vi "SwerveJoystickLogic.vi"(8 "Gyro":dbl, 9 "Ackerman":bool, 10 "Joystick Axes":dbl[](array[numeric])) -> (2 "Speeds":dbl[](array[numeric]), 3 "Angles":dbl[](array[numeric]))   [LabVIEW 2018]
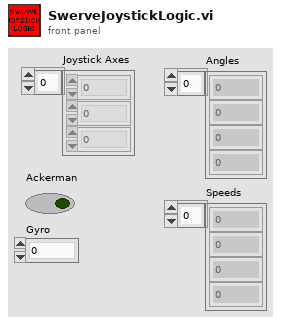
[diagram p1: front panel]
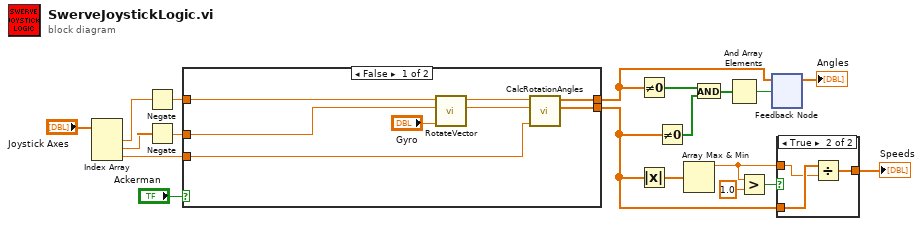
[diagram p0: block diagram]
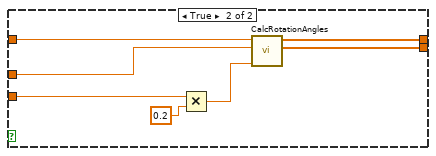
[diagram p3: hidden frame]
diagram:
  n1 = Index Array(array="Joystick Axes") -> (element #1=w6:dbl, element #2=w4:dbl, element #3=w3:dbl)  [unwired: 3 in]
  n2 = Negate(x=w6) -> (-x=w7:dbl)
  n3 = Negate(x=w4) -> (-x=w5:dbl)
  n4 = case shown="False" "Ackerman" {
    tunnel: [w27 w31] -> w14
    tunnel: w7 -> [w25 w34]
    tunnel: w5 -> [w24 w33]
    tunnel: w3 -> [w21 w29]
    tunnel: [w26 w32] -> w10
    frame False {
      n5 = call "RotateVector.vi"("Angle"="Gyro", "Y"=w24, "X"=w25) -> ("Y'"=w22:dbl, "X'"=w23:dbl)  [unwired: 6 in]
      n6 = call "CalcRotationAngles.vi"("ZAxis"=w21, "YAxis"=w22, "XAxis"=w23) -> ("Speeds"=w27:dbl[], "Angles"=w26:dbl[])  [unwired: 7 in]
    }
    frame True {
      n7 = Multiply(x=w29, y=0.2 ("x")) -> (x*y=w30:dbl)
      n8 = call "CalcRotationAngles.vi"("ZAxis"=w30, "YAxis"=w33, "XAxis"=w34) -> ("Speeds"=w31:dbl[], "Angles"=w32:dbl[])  [unwired: 7 in]
    }
  }
  n9 = Not Equal To 0?(x=w10) -> (x != 0?=w12:bool[])
  n10 = Absolute Value(x=w14) -> (abs(x)=w16:dbl[])
  n11 = Not Equal To 0?(x=w14) -> (x != 0?=w11:bool[])
  n12 = Array Max & Min(array=w16) -> (max value=w17:dbl)  [unwired: 3 out]
  n13 = And(x=w12, y=w11) -> (x .and. y?=w15:bool[])
  n14 = And Array Elements(Boolean array=w15) -> (logical AND=w9:bool)
  n15 = Greater?(x=w17, y=1.0) -> (0:w19:bool)
  n16 = feedback #1() -> (→"Angles":dbl[])  [unwired: 1 in]
  n17 = feedback-in #1(w10, w9) -> ()
  n18 = case shown="True" w19 {
    tunnel: w14 -> [w35 w38]
    tunnel: w17 -> [_ w37]
    tunnel: [w35 w36] -> w8
    frame False {
    }
    frame True {
      n19 = Divide(x=w38, y=w37) -> (x/y=w36:dbl[])
    }
  }
  "Speeds" <- w8
